vi "Pump Close SV.vi"(8 "error in (no error)":errorcluster, 10 "Process Name":string="Flow Module 1", 11 "State Cluster in":T1={"Pump Module Config"={"GUID"="", "Drop Coords"={"Horizontal"=0, "Vertical"=0}, "Process Name"="", "Settings"={"Cycle Period"=500.0, "Ismatech"={"VISA resource name"="", "Simulated?"=TRUE, "Pump Number"=1.0, "Reverse?"=FALSE}, "Masterflex"={"VISA resource name"="", "Simulated?"=TRUE, "Pump Number"=1.0, "Reverse?"=FALSE}, "Manual Entry"=0.0, "VICI Settings"={"VISA resource name"="", "Simulated?"=TRUE, "Pump Number"=0.0, "Reverse?"=FALSE}, "Output Device"=enum."Default"}, "Load Count"=0}, "State"=enum."Idle", "Start Time"=timestamp(0 s since 1904-01-01), "Current Time"=timestamp(0 s since 1904-01-01), "First Iteration"=FALSE, "Data"={"Pump Speed"=0.0}, "Process Name"="", "Pump On?"=FALSE} {"Pump Module Config"."Settings"."VICI Settings"."Pump Number" min=1.0 max=20.0 step=1.0; "Pump Module Config"."Settings"."Masterflex"."Pump Number" min=1.0 max=20.0 step=1.0; "Pump Module Config"."Settings"."Ismatech"."Pump Number" min=1.0 max=20.0 step=1.0}) -> (0 "error out":errorcluster, 3 "State Cluster out":T1={"Pump Module Config"={"GUID"="", "Drop Coords"={"Horizontal"=0, "Vertical"=0}, "Process Name"="", "Settings"={"Cycle Period"=500.0, "Ismatech"={"VISA resource name"="", "Simulated?"=TRUE, "Pump Number"=1.0, "Reverse?"=FALSE}, "Masterflex"={"VISA resource name"="", "Simulated?"=TRUE, "Pump Number"=1.0, "Reverse?"=FALSE}, "Manual Entry"=0.0, "VICI Settings"={"VISA resource name"="", "Simulated?"=TRUE, "Pump Number"=0.0, "Reverse?"=FALSE}, "Output Device"=enum."VICI M50"}, "Load Count"=0}, "State"=enum."Idle", "Start Time"=timestamp(0 s since 1904-01-01), "Current Time"=timestamp(0 s since 1904-01-01), "First Iteration"=FALSE, "Data"={"Pump Speed"=0.0}, "Process Name"="", "Pump On?"=FALSE} {"Pump Module Config"."Settings"."VICI Settings"."Pump Number" min=1.0 max=20.0 step=1.0; "Pump Module Config"."Settings"."Masterflex"."Pump Number" min=1.0 max=20.0 step=1.0; "Pump Module Config"."Settings"."Ismatech"."Pump Number" min=1.0 max=20.0 step=1.0})   [LabVIEW 2021, in "Pump Module.lvlib"]
uses:
  Pump Module.lvlib
  Shared Variables/Dynamic Shared Variables.lvlib
  Pump Module Settings Cluster.ctl
  Pump Module State Cluster.ctl
  Ismatec ISM 831C/Controls/Ismatech Settings Cluster.ctl
  Masterflex 7550-30/Controls/Settings Cluster.ctl
  Masterflex 7550-30/Masterflex 7550-30.lvlib
  Measure Instrument/PID 2 Output Enum.ctl
  VICI M50/VICI Settings.ctl
  <vilib>/Utility/miscctls.llb/LVPoint32TypeDef.ctl
  Pump Module Config Cluster.ctl
  Measure Instrument/State Enum.ctl
  Measure Instrument/Feed Module Engine.lvlib
panel:
  # "Output Instruments"
  # "Output Instruments"
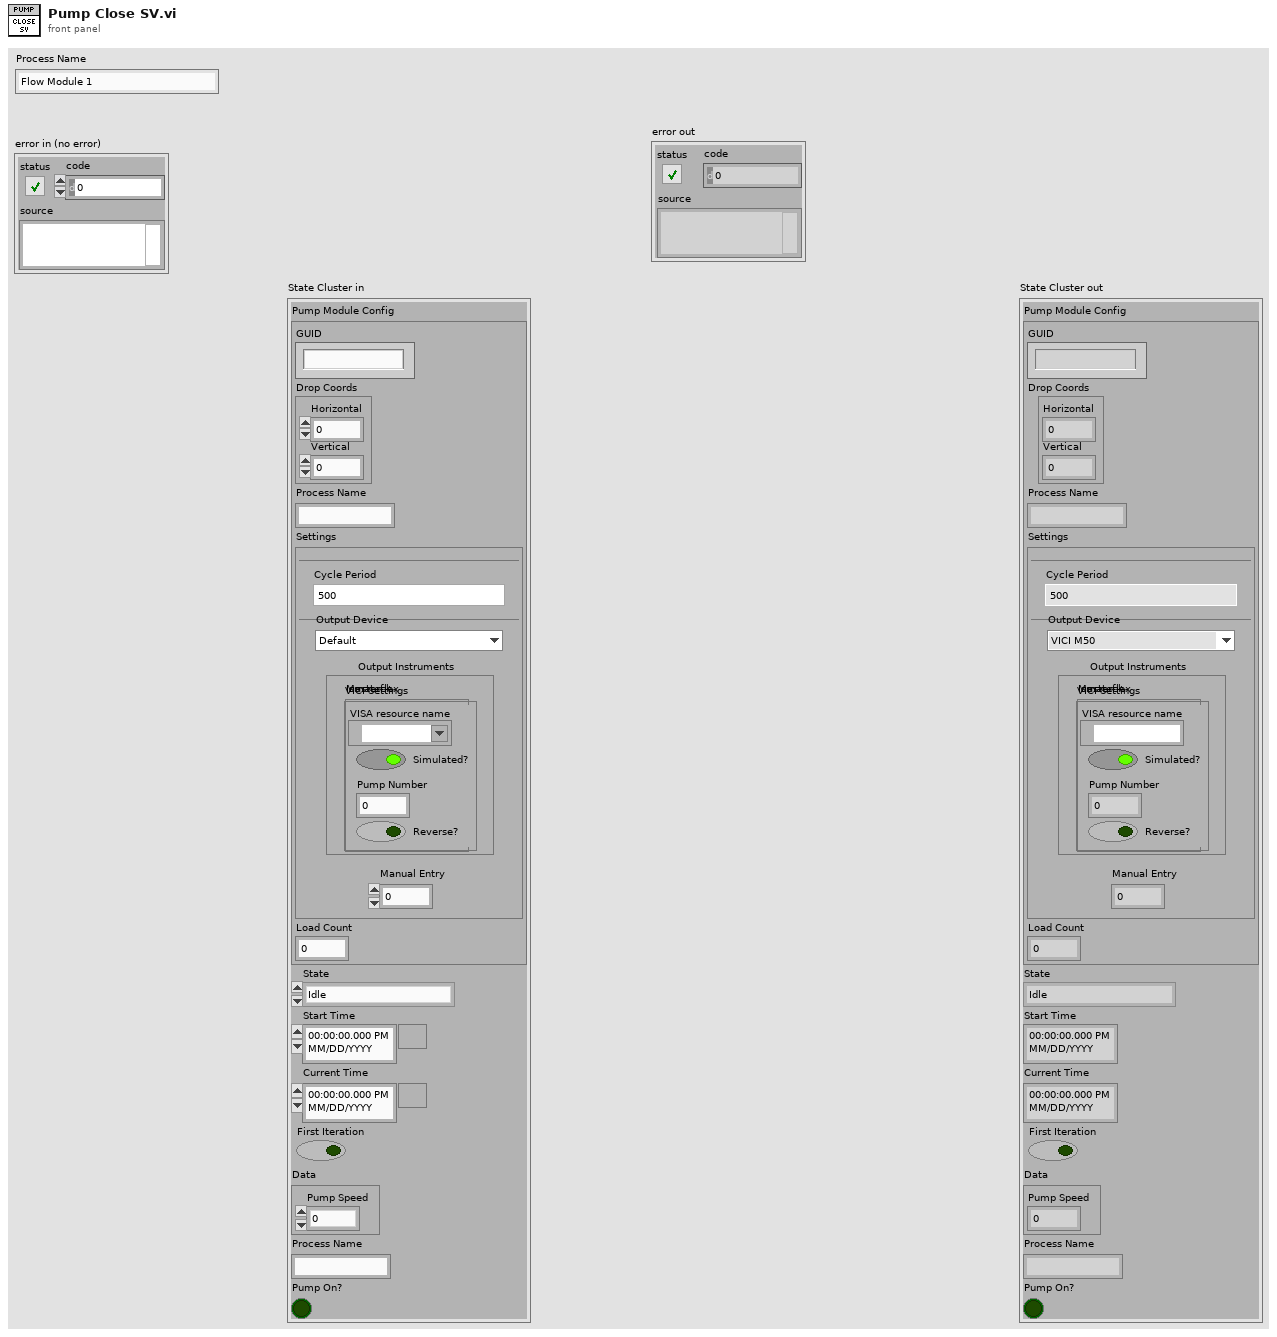
[diagram p1: front panel]
types:
  T1 = typedef "Pump Module.lvlib/Pump Module State Cluster.ctl" = cluster{"Pump Module Config":T2, "State":T9, "Start Time":timestamp, "Current Time":timestamp, "First Iteration":bool, "Data":cluster{"Pump Speed":dbl}, "Process Name":string, "Pump On?":bool}
  T2 = typedef "Pump Module.lvlib/Pump Module Config Cluster.ctl" = cluster{"GUID":string, "Drop Coords":T3, "Process Name":string, "Settings":T4, "Load Count":i32}
  T3 = typedef "LVPoint32TypeDef.ctl" = cluster{"Horizontal":i32, "Vertical":i32}
  T4 = typedef "Pump Module.lvlib/Pump Module Settings Cluster.ctl" = cluster{"Cycle Period":dbl, "Ismatech":T5, "Masterflex":T6, "Manual Entry":dbl, "VICI Settings":T7, "Output Device":T8}
  T5 = typedef "Ismatec ISM 831C.lvlib/Ismatech Settings Cluster.ctl" = cluster{"VISA resource name":refnum<visa-resource-name>, "Simulated?":bool, "Pump Number":dbl, "Reverse?":bool}
  T6 = typedef "Masterflex 7550-30.lvlib/Settings Cluster.ctl" = cluster{"VISA resource name":refnum<visa-resource-name>, "Simulated?":bool, "Pump Number":dbl, "Reverse?":bool}
  T7 = typedef "VICI Settings.ctl" = cluster{"VISA resource name":refnum<visa-resource-name>, "Simulated?":bool, "Pump Number":dbl, "Reverse?":bool}
  T8 = typedef "PID 2 Output Enum.ctl" = enum16{"Default", "Ismatec ISM 4308", "Ismatec ISM 831C", "Masterflex 7550-30", "VICI M6", "VICI M50", "Tacmina QI", "KNF SIMDOS", "ASIA Type C", "FLOM UI-22-11", "SSI PR/LD", "SSI P40", "Masterflex 75211-70"}
  T9 = typedef "Feed Module.lvlib/Feed Module Engine.lvlib/State Enum.ctl" = enum16{"Measuring", "Idle", "Paused"}
  T10 = typedef "Pump Module.lvlib/Pump Module Shared Variable Cluster.ctl" = cluster{"PID 1 Process Variable":string, "PID 1 Output":string, "PID 1 Setpoint":string, "PID 1 Setpoint SV refnum":refnum<k21>, "PID 1 Process Variable SV refnum":refnum<k21>, "PID 1 Output SV refnum":refnum<k21>}
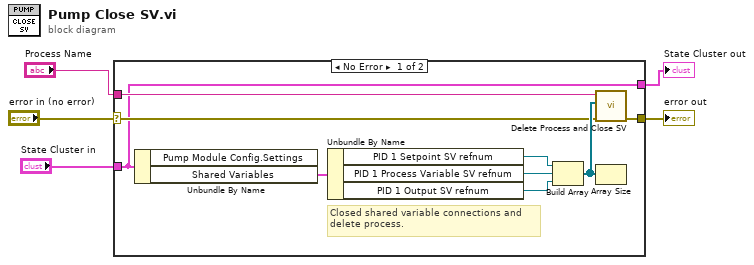
[diagram p0: block diagram]
diagram:
  n1 = case shown="No Error" "error in (no error)" {
    selector: "error in (no error)" -> [w8 w16]
    tunnel: "Process Name" -> [w13 _]
    tunnel: [w7 w16] -> w3
    tunnel: "State Cluster in" -> [w6 w15]
    tunnel: [w6 w15] -> w1
    frame No Error {
      # "Closed shared variable connections and\ndelete process."
      n2 = Unbundle By Name(w6) -> ("Shared Variables"=w14:T10)  [unwired: 1 out]
      n3 = Unbundle By Name(w14) -> ("PID 1 Setpoint SV refnum"=w12:refnum<k21>, "PID 1 Process Variable SV refnum"=w11:refnum<k21>, "PID 1 Output SV refnum"=w10:refnum<k21>)
      n4 = Build Array(w12, w11, w10) -> (w9:refnum<k21>[])
      n5 = call "Delete Process and Close SV.vi"("error in (no error)"=w8, "Array"=w9, "process name"=w13) -> ("error out"=w7:errorcluster)  [unwired: 8 in]
      n6 = Array Size(array=w9) -> ()  [unwired: 1 out]
    }
    frame Error {
    }
  }
  "error out" <- w3
  "State Cluster out" <- w1
